vi "UserLogin.vi"() -> ()   [LabVIEW 2023]
uses:
  <vilib>/userDefined/High Color/IMAQdx.ctl
  <vilib>/vision/driver/NI_Vision_Acquisition_Software.lvlib
panel:
  in  "Plik wyjsciowy 2":path=path "f:/test.jpg"
  in  "Zapisz 2":bool
  in  "Tab Control":enum32{"Page 1", "Page 2", "Page 3"}(tab)
  in  "stop 2":bool
  out "Image 3":T1(plugin-control) caption="Image"
  in  "Password":string
  in  "User":string
  in  "Refresh Button":bool
  out "Answer":dbl
  in  "Numeric 2":dbl
  in  "Numeric":dbl
  in  "Stop Button":bool
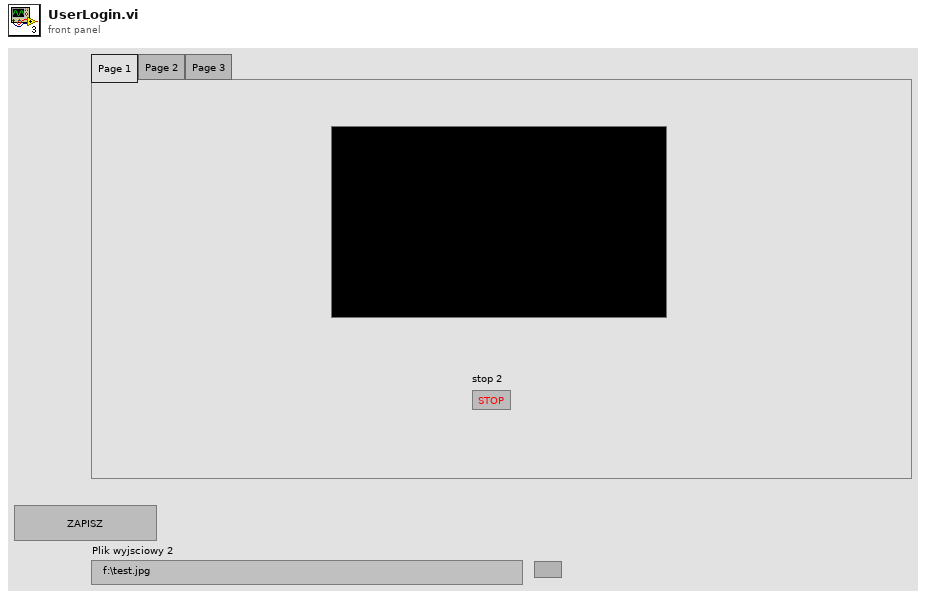
[diagram p1: front panel]
types:
  T1 = typedef "IMAQ Image.ctl" = refnum<image>
  T2 = typedef "IMAQdx.ctl" = refnum<k21>
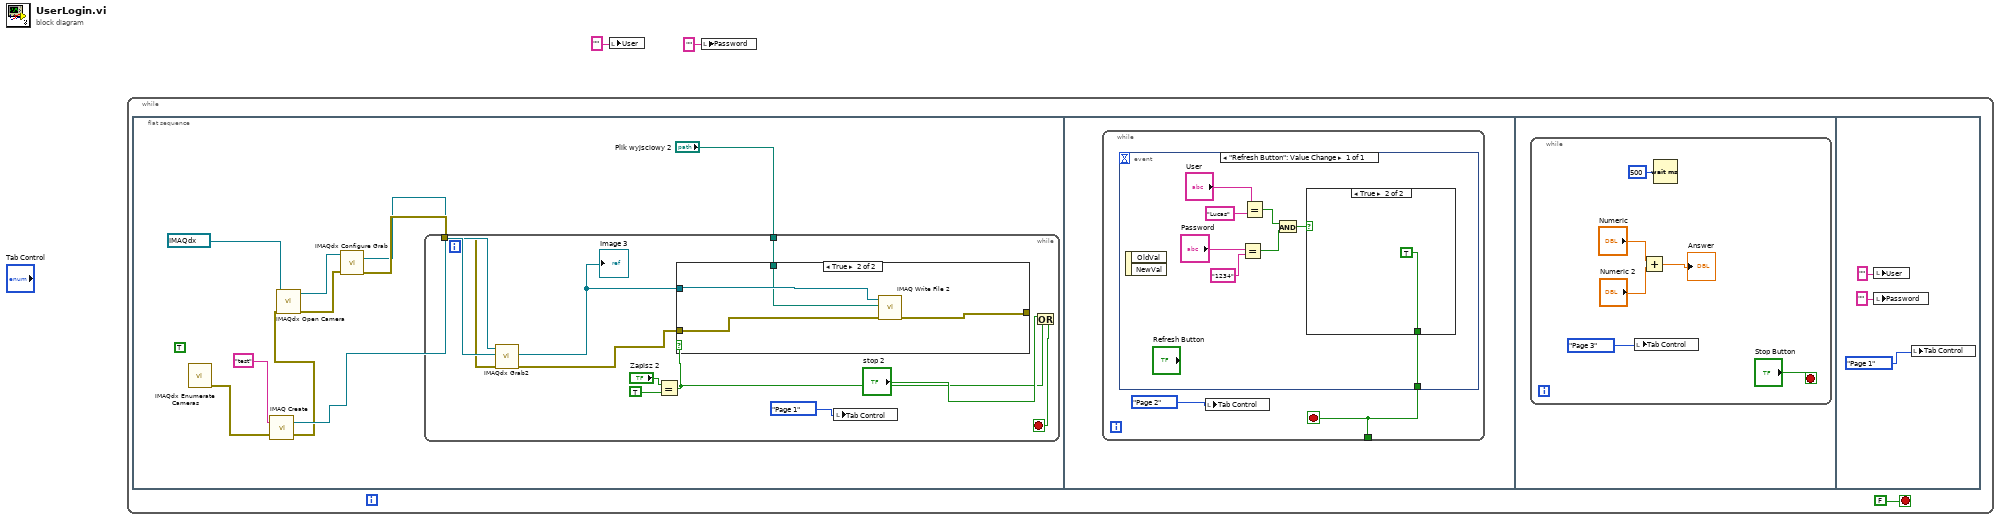
[diagram p0: block diagram]
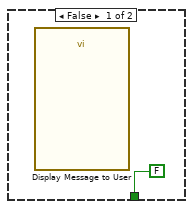
[diagram p3: hidden frame]
diagram:
  n1 = while {
    stop <- FALSE stop-if-true
    n2 = flat-sequence {
      frame #0 {
        (unwired) TRUE ("Connected Only? (Yes)")
        n3 = call <vilib>:"IMAQdx Enumerate Cameras.vi"() -> ("error out"=w6:errorcluster)  [unwired: 10 in, 1 out]
        n4 = call "IMAQ Create"("Image Name"="test", "error in (no error)"=w6) -> ("New Image"=w8:T1, "error out"=w7:errorcluster)  [unwired: 2 in, 1 out]
        n5 = call <vilib>:"IMAQdx Open Camera.vi"("error in"=w7, "Session In"=T2 "cam0") -> ("error out"=w10:errorcluster, "Session Out"=w9:T2)  [unwired: 1 in, 7 out]
        n6 = call <vilib>:"IMAQdx Configure Grab.vi"("error in"=w10, "Session In"=w9) -> ("error out"=w13:errorcluster, "Session Out"=w12:T2)  [unwired: 8 in]
        n7 = while {
          tunnel: w8 -> [w22]
          tunnel: "Plik wyjsciowy 2" -> [w19]
          tunnel: w12 -> [w17]
          tunnel: w13 -> [w16]
          stop <- w20 stop-if-true
          n8 = call <vilib>:"IMAQdx Grab2.vi"("error in"=w16, "Image In"=w22, "Session In"=w17) -> ("error out"=w23:errorcluster, "Image Out"=w18:T1)  [unwired: 5 in, 2 out]
          "Image 3" <- w18
          n9 = Equal?(x="Zapisz 2", y=TRUE) -> (x = y?=w15:bool)
          n10 = case shown="True" w15 {
            tunnel: w23 -> [w26 w30]
            tunnel: w18 -> [_ w29]
            tunnel: w19 -> [_ w28]
            tunnel: [w26 w27] -> _
            frame False {
            }
            frame True {
              n11 = call-poly "IMAQ Write File 2"("error in (no error)"=w30, "File Path"=w28, "Image"=w29) -> ("error out"=w27:errorcluster)  [unwired: 2 in, 6 out]
            }
          }
          n12 = local write "Tab Control"(enum32{"Page 1", "Page 2", "Page 3"}."Page 1" ("Tab Control")) -> ()
          n13 = Or(x="stop 2", y=w15) -> (x .or. y?=w20:bool)
        }
      }
      frame #1 {
        n14 = while {
          tunnel: [w32] -> _
          stop <- w32 stop-if-true
          n15 = event shown="[0] \"Refresh Button\": Value Change" {
            selector: _ -> [_]
            dyn-events: _ -> [_]
            timeout: _ -> [_]
            tunnel: [w33] -> w32
            event "Refresh Button": Value Change {
              n16 = event-data() -> ()  [unwired: 1 in, 2 out]
              n17 = Equal?(x="Password", y="1234" ("x")) -> (x = y?=w35:bool)
              n18 = Equal?(x="User", y="Lucas") -> (x = y?=w36:bool)
              n19 = And(x=w36, y=w35) -> (x .and. y?=w34:bool)
              n20 = case shown="True" w34 {
                tunnel: [FALSE TRUE] -> w33
                frame False {
                  n21 = call "Display Message to User"() -> ()  [unwired: 10 in, 2 out]
                }
                frame True {
                }
              }
            }
          }
          n22 = local write "Tab Control"(enum32{"Page 1", "Page 2", "Page 3"}."Page 2" ("Tab Control")) -> ()
        }
      }
      frame #2 {
        n23 = while {
          stop <- "Stop Button" stop-if-true
          n24 = local write "Tab Control"(enum32{"Page 1", "Page 2", "Page 3"}."Page 3" ("Tab Control")) -> ()
          n25 = Add(x="Numeric", y="Numeric 2") -> (x+y=→"Answer":dbl)
          n26 = Wait (ms)(milliseconds to wait=u32 500) -> ()  [unwired: 1 out]
        }
      }
      frame #3 {
        n27 = local write "User"("" ("User")) -> ()
        n28 = local write "Password"("" ("Password")) -> ()
        n29 = local write "Tab Control"(enum32{"Page 1", "Page 2", "Page 3"}."Page 1" ("Tab Control")) -> ()
      }
    }
  }
  n30 = local write "User"("" ("User")) -> ()
  n31 = local write "Password"("" ("Password")) -> ()
